vi "Error code find.vi"(3 "Table Control":string[][](table)) -> (1 "Error code":i32)   [LabVIEW 2015]
panel:
  out "Error":string
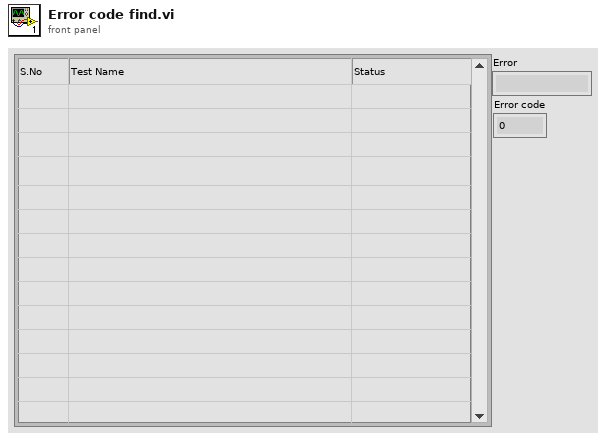
[diagram p1: front panel]
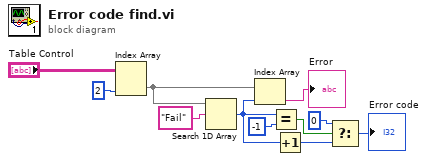
[diagram p0: block diagram]
diagram:
  n1 = Index Array(array="Table Control", index (col)=2 ("disabled index (col)")) -> (element=w8:string[])  [unwired: 1 in]
  n2 = Search 1D Array(1D array=w8, element="Fail") -> (index of element=w3:i32)  [unwired: 1 in]
  n3 = Index Array(array=w8, index=w3) -> (element=→"Error":string)
  n4 = Equal?(x=w3, y=-1) -> (x = y?=w5:bool)
  n5 = Increment(x=w3) -> (x+1=w1:i32)
  n6 = Select(t=0 ("y"), s=w5, f=w1) -> (s? t:f=→"Error code":i32)
